vi "Step 5.vi"(8 "error in (no error)":errorcluster, 11 "HeatUp Data in":string[][](array[string])) -> (0 "error out":errorcluster, 2 "Tank Gradient":dbl, 3 "Max Temp Drift":dbl, 4 "Tank Gradient Data":string[][](array[string]))   [LabVIEW 2016]
uses:
  <vilib>/Utility/error.llb/DialogType.ctl
panel:
  out "Heat Up Data with Only Selected Columns":string[][](array[string])
  out "Gradient Row":dbl[](array[numeric])
  out "Array 4":string[][](array[string])
  out "Array 3":string[][](array[string])
  out "3 Min Time":dbl
  out "Start Time":dbl
  out "Setpoint-TCAvg":dbl[](graph)
  out "Deleted Rows":i32[](array[numeric])
  out "T2-Setpoint":dbl[](graph)
  out "Setpoint":dbl[](graph)
  out "T2":dbl[](graph)
  out "Lower Heat Source Cutout":string[][](array[string])
  # "Data with Stripped Header"
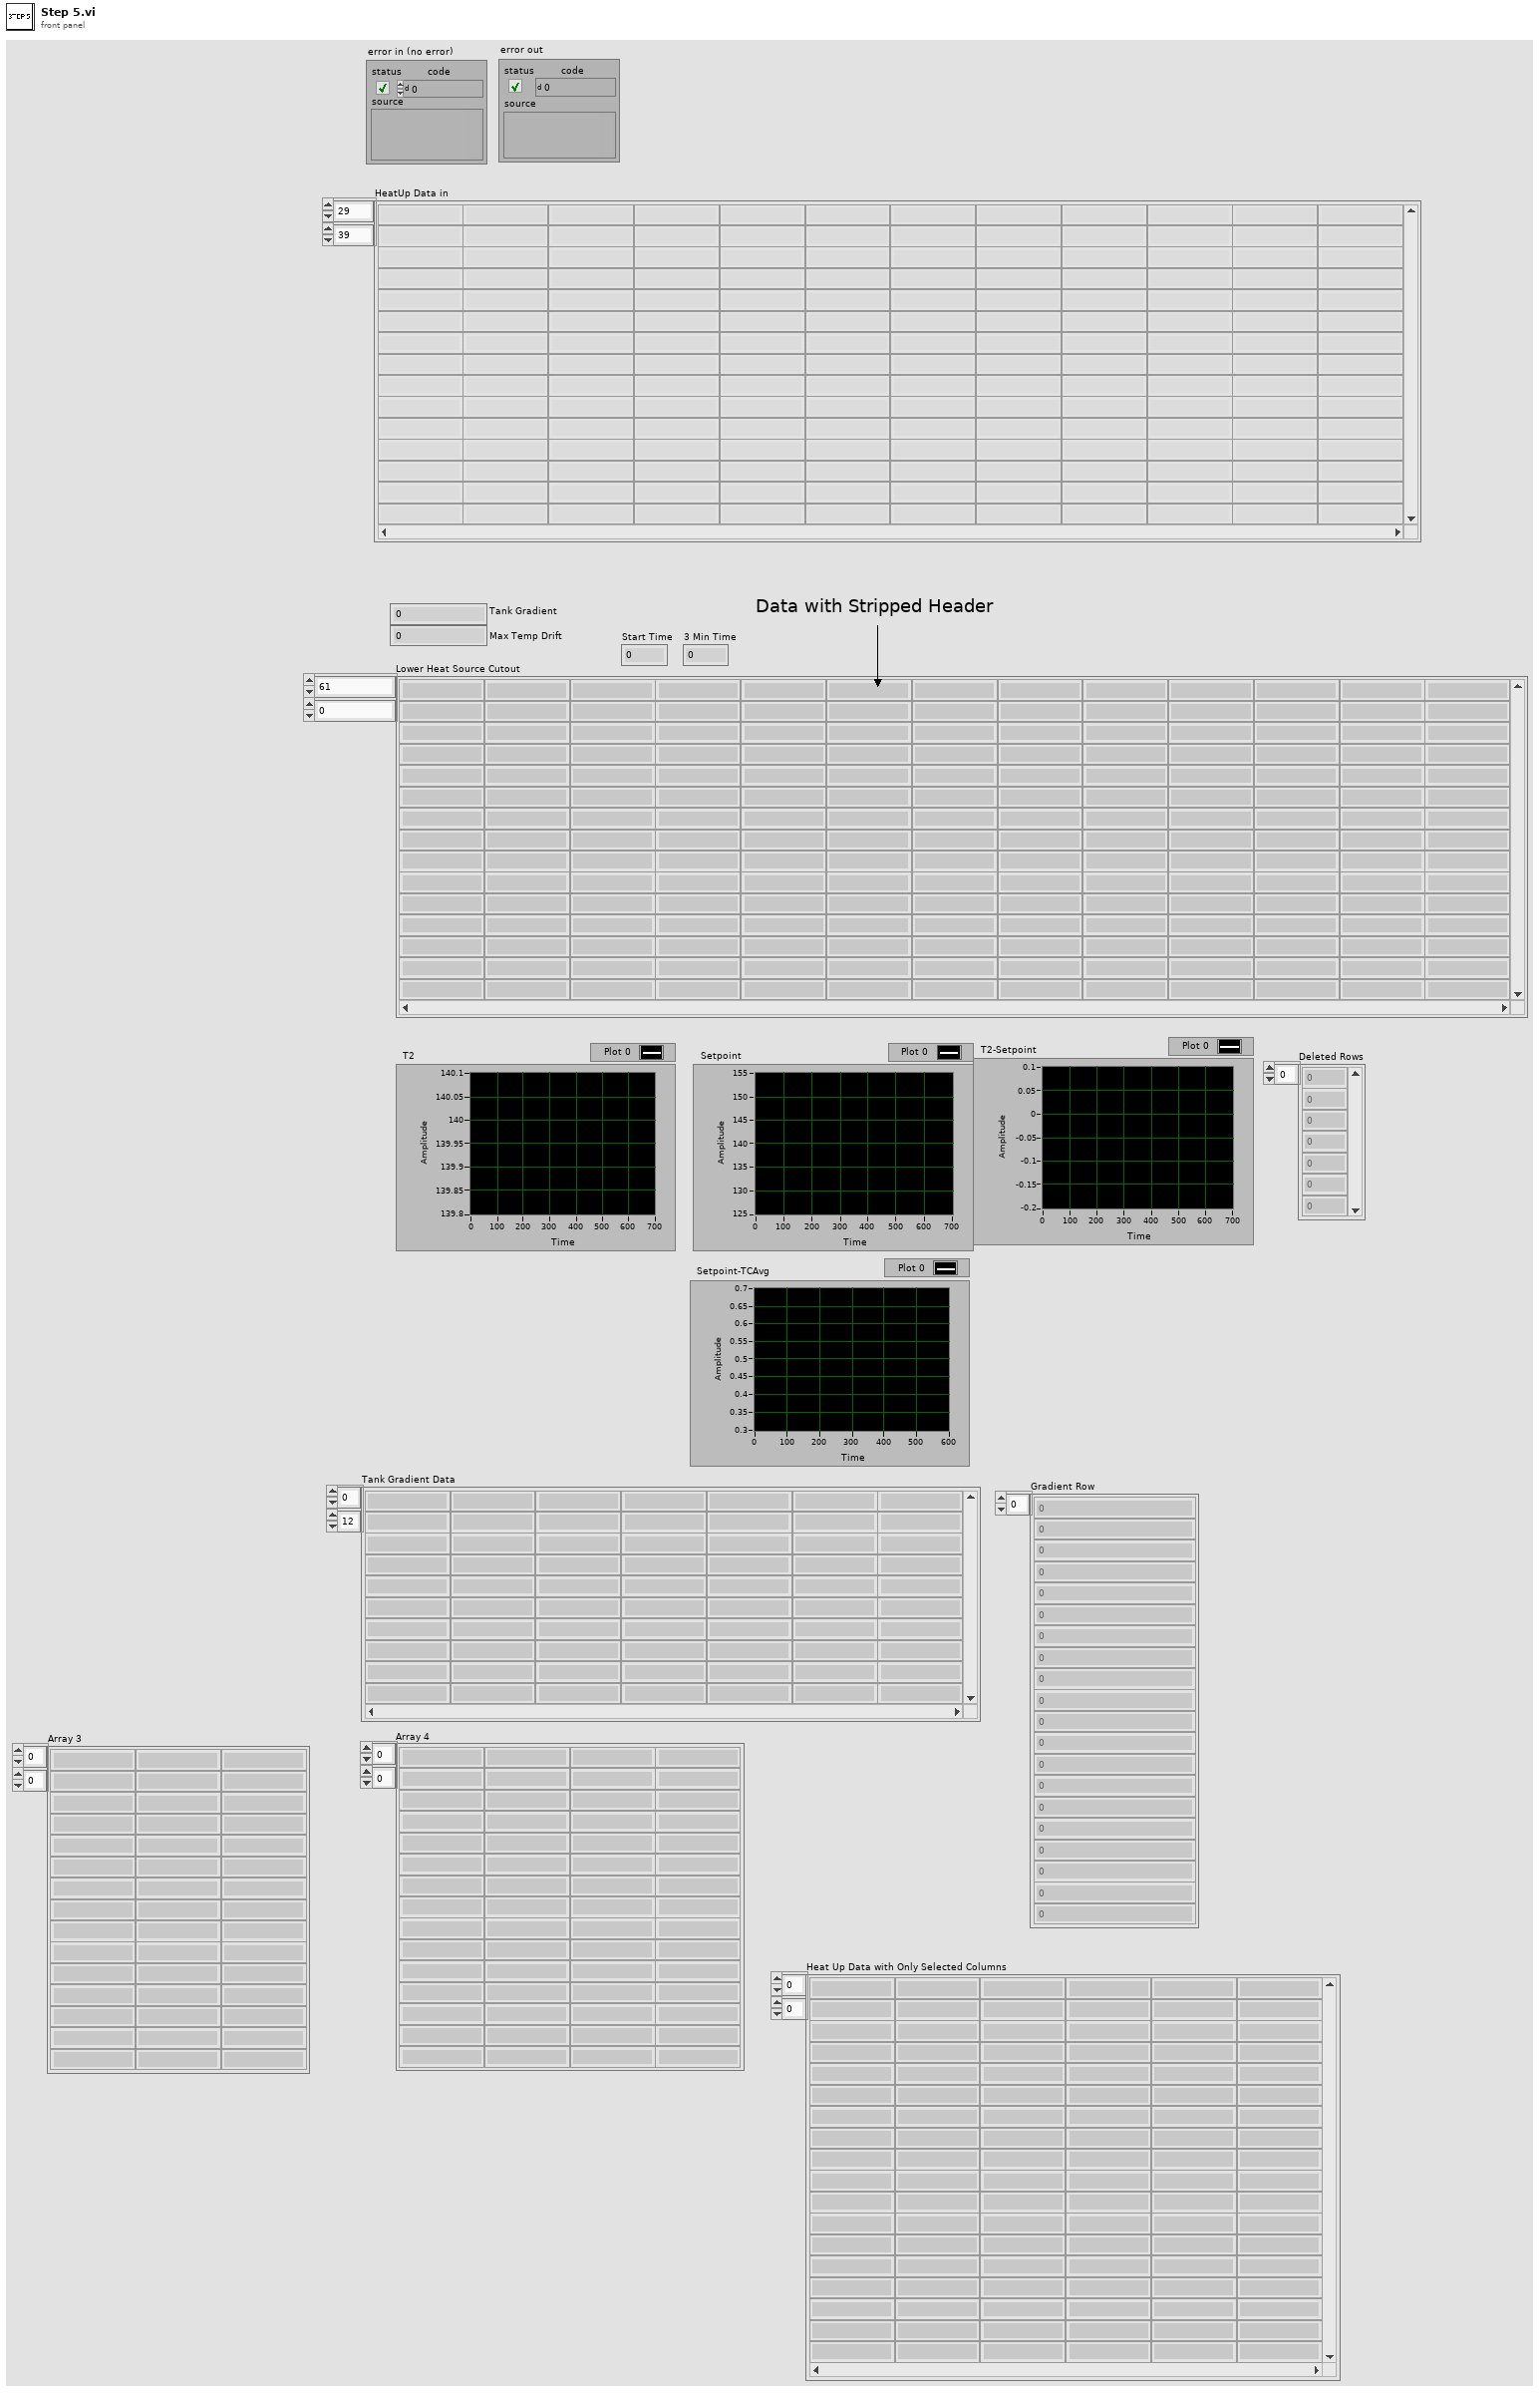
[diagram p1: front panel]
types:
  T1 = typedef "DialogType.ctl" = u16
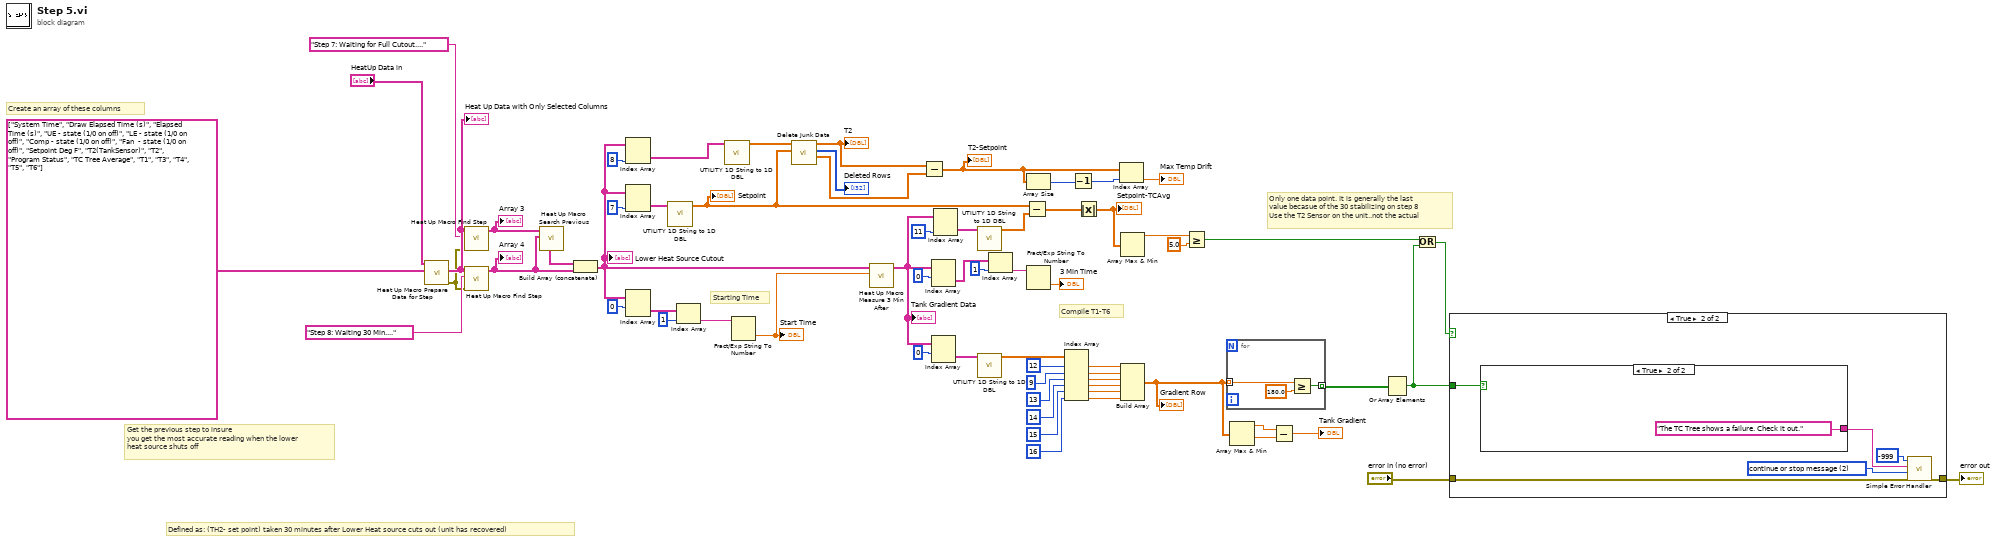
[diagram p0: block diagram]
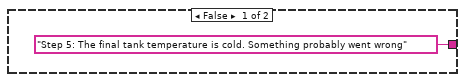
[diagram p3: hidden frame]
diagram:
  # "Compile T1-T6"
  # "Get the previous step to insure \nyou get the most accurate reading when the lower\nheat source shuts off"
  # "Only one data point. It is generally the last \nvalue becasue of the 30 stabilizing on step 8\nUse the T2 Sensor on the unit..not the actual"
  # "Starting Time"
  # "Defined as: (TH2- set point) taken 30 minutes after Lower Heat source cuts out (unit has recovered)"
  # "Create an array of these columns"
  n1 = call "Heat Up Macro Prepare Data for Step.vi"("Columns Too Search For"=string[] ["System Time", "Draw Elapsed Time (s)", "Elapsed Time (s)", "UE - state (1/0 on off)", "LE - state (1/0 on off)", "Comp - state (1/0 on off)", "Fan  - state (1/0 on off)", "Setpoint Deg F", "T2(TankSensor)", "T2", "Program Status", "TC Tree Average", "T1", "T3", "T4", "T5", "T6"], "HeatUp Raw Data Input"="HeatUp Data in") -> ("Error Out"=w7:errorcluster, "Heat Up Data with Only Selected Columns"=w10:string[][])  [unwired: 8 in]
  "Heat Up Data with Only Selected Columns" <- w10
  n2 = call "Heat Up Macro Find Step.vi"("Error In"=w7, "Search For Step Name"="Step 7: Waiting for Full Cutout...." ("y"), "Heat Up Data with Only Selected Columns"=w10) -> ("Filtered Array"=w8:string[][])  [unwired: 6 in, 2 out]
  "Array 3" <- w8
  n3 = call "Heat Up Macro Find Step.vi"("Error In"=w7, "Search For Step Name"="Step 8: Waiting 30 Min...." ("y"), "Heat Up Data with Only Selected Columns"=w10) -> ("Filtered Array"=w43:string[][])  [unwired: 6 in, 2 out]
  "Array 4" <- w43
  n4 = call "Heat Up Macro Search Previous.vi"("Step 8"=w43, "Step 7"=w8) -> ("Output Array"=w44:string[][])  [unwired: 2 in, 7 out]
  n5 = Build Array (concatenate)(w44, w43) -> (w42:string[][])
  "Lower Heat Source Cutout" <- w42
  n6 = Index Array(array=w42, index (col)=8 ("disabled index (col)")) -> (element=w64:string[])  [unwired: 1 in]
  n7 = Index Array(array=w42, index (col)=7 ("disabled index (col)")) -> (element=w63:string[])  [unwired: 1 in]
  n8 = Index Array(array=w42, index (row)=0) -> (element=w57:string[])  [unwired: 1 in]
  n9 = call "UTILITY 1D String to 1D DBL.vi"("Save Data"=w63) -> ("DBL"=w51:dbl[])  [unwired: 10 in]
  "Setpoint" <- w51
  n10 = Index Array(array=w57, index=1) -> (element=w55:string)
  n11 = call "UTILITY 1D String to 1D DBL.vi"("Save Data"=w64) -> ("DBL"=w62:dbl[])  [unwired: 10 in]
  n12 = Fract/Exp String To Number(string=w55) -> (number=w54:dbl)  [unwired: 3 in, 1 out]
  "Start Time" <- w54
  n13 = call "Delete Junk Data.vi"("DAQ Array"=w51, "Newfi Input Array"=w62) -> ("DAQ Array Output"=w59:dbl[], "Deleted Rows"=→"Deleted Rows":i32[], "Data"=w61:dbl[])  [unwired: 7 in]
  "T2" <- w61
  n14 = call "Heat Up Macro Measure 3 Min After.vi"("Start Time"=w54, "Array in"=w42) -> ("Array out"=w16:string[][])  [unwired: 9 in]
  "Tank Gradient Data" <- w16
  n15 = Subtract(x=w61, y=w59) -> (x-y=w41:dbl[])
  "T2-Setpoint" <- w41
  n16 = Index Array(array=w16, index (row)=0) -> (element=w18:string[])  [unwired: 1 in]
  n17 = Index Array(array=w16, index (row)=0) -> (element=w36:string[])  [unwired: 1 in]
  n18 = Index Array(array=w16, index (col)=11 ("disabled index (col)")) -> (element=w52:string[])  [unwired: 1 in]
  n19 = call "UTILITY 1D String to 1D DBL.vi"("Save Data"=w52) -> ("DBL"=w45:dbl[])  [unwired: 10 in]
  n20 = call "UTILITY 1D String to 1D DBL.vi"("Save Data"=w36) -> ("DBL"=w35:dbl[])  [unwired: 10 in]
  n21 = Index Array(array=w18, index=1) -> (element=w15:string)
  n22 = Subtract(x=w51, y=w45) -> (x-y=w50:dbl[])
  n23 = Array Size(array=w41) -> (size(s)=w39:i32)
  n24 = Fract/Exp String To Number(string=w15) -> (number=→"3 Min Time":dbl)  [unwired: 3 in, 1 out]
  n25 = Index Array(array=w35, index #1=12 ("index"), index #2=9 ("index"), index #3=13 ("index"), index #4=14 ("index"), index #5=15 ("index"), index #6=16 ("index")) -> (element #1=w28:dbl, element #2=w27:dbl, element #3=w26:dbl, element #4=w25:dbl, element #5=w24:dbl, element #6=w23:dbl)
  n26 = Decrement(x=w39) -> (x-1=w38:i32)
  n27 = Absolute Value(x=w50) -> (abs(x)=w49:dbl[])
  "Setpoint-TCAvg" <- w49
  n28 = Index Array(array=w41, index=w38) -> (element=→"Max Temp Drift":dbl)
  n29 = Array Max & Min(array=w49) -> (max value=w48:dbl)  [unwired: 3 out]
  n30 = Build Array(w28, w27, w26, w25, w24, w23) -> (w6:dbl[])
  "Gradient Row" <- w6
  n31 = Greater Or Equal?(x=w48, y=5.0) -> (x >= y?=w4:bool)
  n32 = for {
    tunnel: w6 -> [w69] mode=indexing
    tunnel: [w67] -> w5 mode=indexing
    n33 = Greater Or Equal?(x=w69, y=180.0) -> (x >= y?=w67:bool)
  }
  n34 = Array Max & Min(array=w6) -> (max value=w22:dbl, min value=w21:dbl)  [unwired: 2 out]
  n35 = Subtract(x=w22, y=w21) -> (x-y=→"Tank Gradient":dbl)
  n36 = Or Array Elements(Boolean array=w5) -> (logical OR=w2:bool)
  n37 = Or(x=w4, y=w2) -> (x .or. y?=w3:bool)
  n38 = case shown="True" w3 {
    tunnel: "error in (no error)" -> [w70 w76]
    tunnel: [w70 w75] -> w46
    tunnel: w2 -> [_ w71]
    frame False {
    }
    frame True {
      w74 = T1 2 items=["no dialog", "OK message", "continue or stop message", "OK message + warnings", "continue/stop + warnings"] ("type of dialog (OK msg:1)")
      n39 = case shown="True" w71 {
        tunnel: ["Step 5: The final tank temperature is cold. Something probably went wrong" ("error source (\" \")") "The TC Tree shows a failure. Check it out." ("error source (\" \")")] -> w73
        frame False {
        }
        frame True {
        }
      }
      n40 = call <vilib>:"Simple Error Handler.vi"("error code (no error:0)"=-999, "error source (\" \")"=w73, "type of dialog (OK msg:1)"=w74, "error in (no error)"=w76) -> ("error out"=w75:errorcluster)  [unwired: 1 in, 4 out]
    }
  }
  "error out" <- w46
